vi "DAQNavi Read (Buffered Counter Pulse Width).vi"(8 "error in (no error)":errorcluster, 9 "number of samples per channel to read":i32=10, 10 "timeout":dbl=10.0, 11 "task in":i32) -> (0 "error out":errorcluster, 2 "data":cluster{"high period":dbl, "low period":dbl}[][](array[cluster]), 3 "task out":i32)   [LabVIEW 2020]
uses:
  DAQNavi_LV.dll
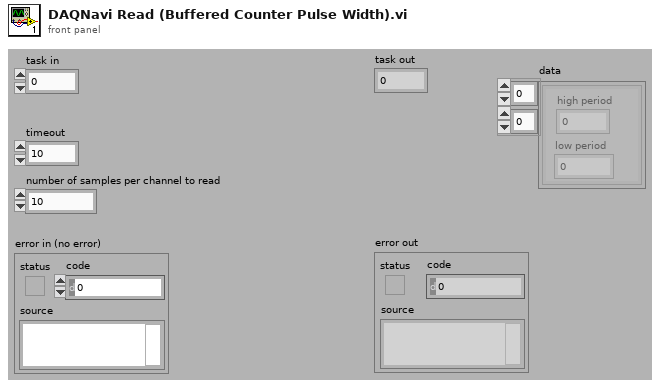
[diagram p1: front panel]
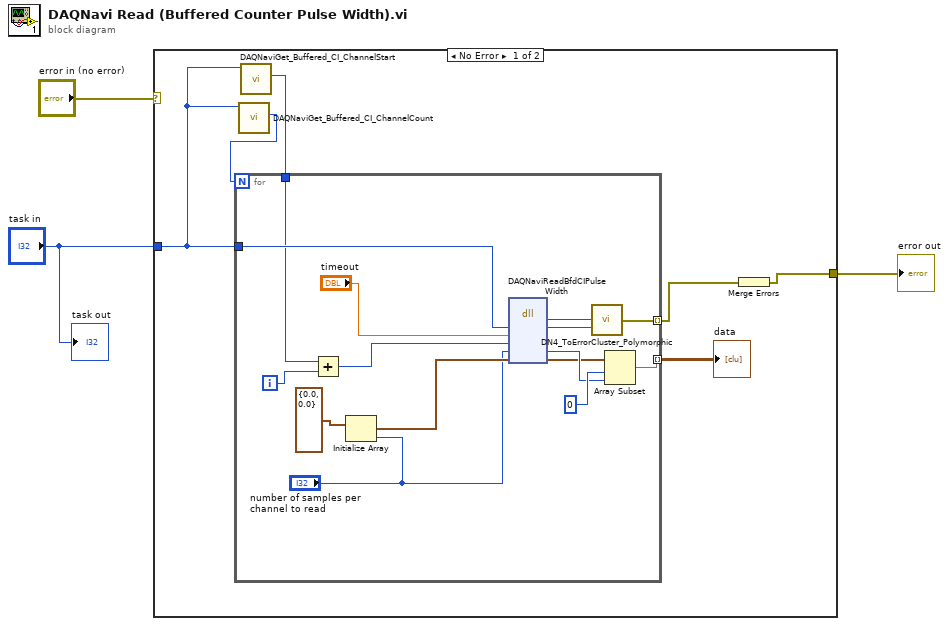
[diagram p0: block diagram]
diagram:
  n1 = case shown="No Error" "error in (no error)" {
    selector: "error in (no error)" -> [_ w25]
    tunnel: "task in" -> [w6 _]
    tunnel: [w8 w25] -> w1
    frame No Error {
      n2 = call "DAQNaviGet_Buffered_CI_ChannelCount.vi"("task in"=w6) -> ("channelCount"=w7:i32)  [unwired: 1 in, 9 out]
      n3 = call "DAQNaviGet_Buffered_CI_ChannelStart.vi"("task in"=w6) -> ("channelStart"=w5:i32)  [unwired: 1 in, 9 out]
      n4 = for {
        N: w7 -> [_]
        tunnel: w6 -> [w24]
        tunnel: [w17] -> w9 mode=indexing
        tunnel: w5 -> [w16]
        tunnel: [w10] -> w4 mode=indexing
        i -> [w20]
        n5 = Add(x=w16, y=w20) -> (x+y=w19:i32)
        n6 = Initialize Array(cluster{dbl, dbl} {0.0, 0.0}, "number of samples per channel to read") -> (w23:cluster{dbl, dbl}[])
        n7 = dll-call lib="DAQNavi_LV.dll" fn="DAQNaviReadBfdCIPulseWidth"("taskID"=w24, "timeout"="timeout", "cntr"=w19, "count"="number of samples per channel to read", "samples"=w23) -> ("return type"=w18:i32, "taskID"=w15:i32, "count"=w12:i32, "samples"=w11:cluster{dbl, dbl}[])  [unwired: 5 in, 2 out]
        n8 = call "DN4_ToErrorCluster_Polymorphic.vi"("task id"=w15, "error code"=w18) -> ("error out"=w17:errorcluster)  [unwired: 3 out]
        n9 = Array Subset(array=w11, index=0, length=w12) -> (w10:cluster{dbl, dbl}[])
      }
      "data" <- w4
      n10 = Merge Errors(w9) -> (w8:errorcluster)
    }
    frame Error {
    }
  }
  "error out" <- w1
  "task out" <- "task in"
